vi "GetClassTemplates.vi"(0 "ClassWriterGOOP400 in":refnum<class "ClassWriterGOOP400.lvclass">, 1 "DerivedFromThisClass(if any)":refnum<vi>, 5 "error in (no error)":errorcluster) -> (14 "ClassWriterGOOP400 out":refnum<class "ClassWriterGOOP400.lvclass">, 15 "Templates":T1[](array[typedef]), 19 "error out":errorcluster)   [LabVIEW 2020, in "ClassWriterGOOP400.lvclass"]
uses:
  <resource>/Framework/Providers/Open_GDS/ClassProviders/Provider_EndevoGOOP400/ClassWriterGOOP400_class/ClassWriterGOOP400.lvclass
  <resource>/Framework/Providers/Open_GDS/ClassProviders/Provider_BaseClassInterface/ClassTemplateType.ctl
  <resource>/Framework/Providers/Open_GDS/ClassProviders/Provider_EndevoGOOP400/Templates/EndevoG4TemplateNames.ctl
  <resource>/Framework/Providers/Open_GDS/ClassProviders/Common/ScriptingFunctions/Scripting_ConnectorPanePatternType.ctl
  <resource>/Framework/Providers/Open_GDS/ClassProviders/Provider_BaseClassInterface/ClassWriter_class/ClassWriter.lvclass
  <resource>/Framework/Providers/Open_GDS/ClassProviders/Provider_LvNativeClass/ClassWriterNative_class/ClassWriterNative.lvclass
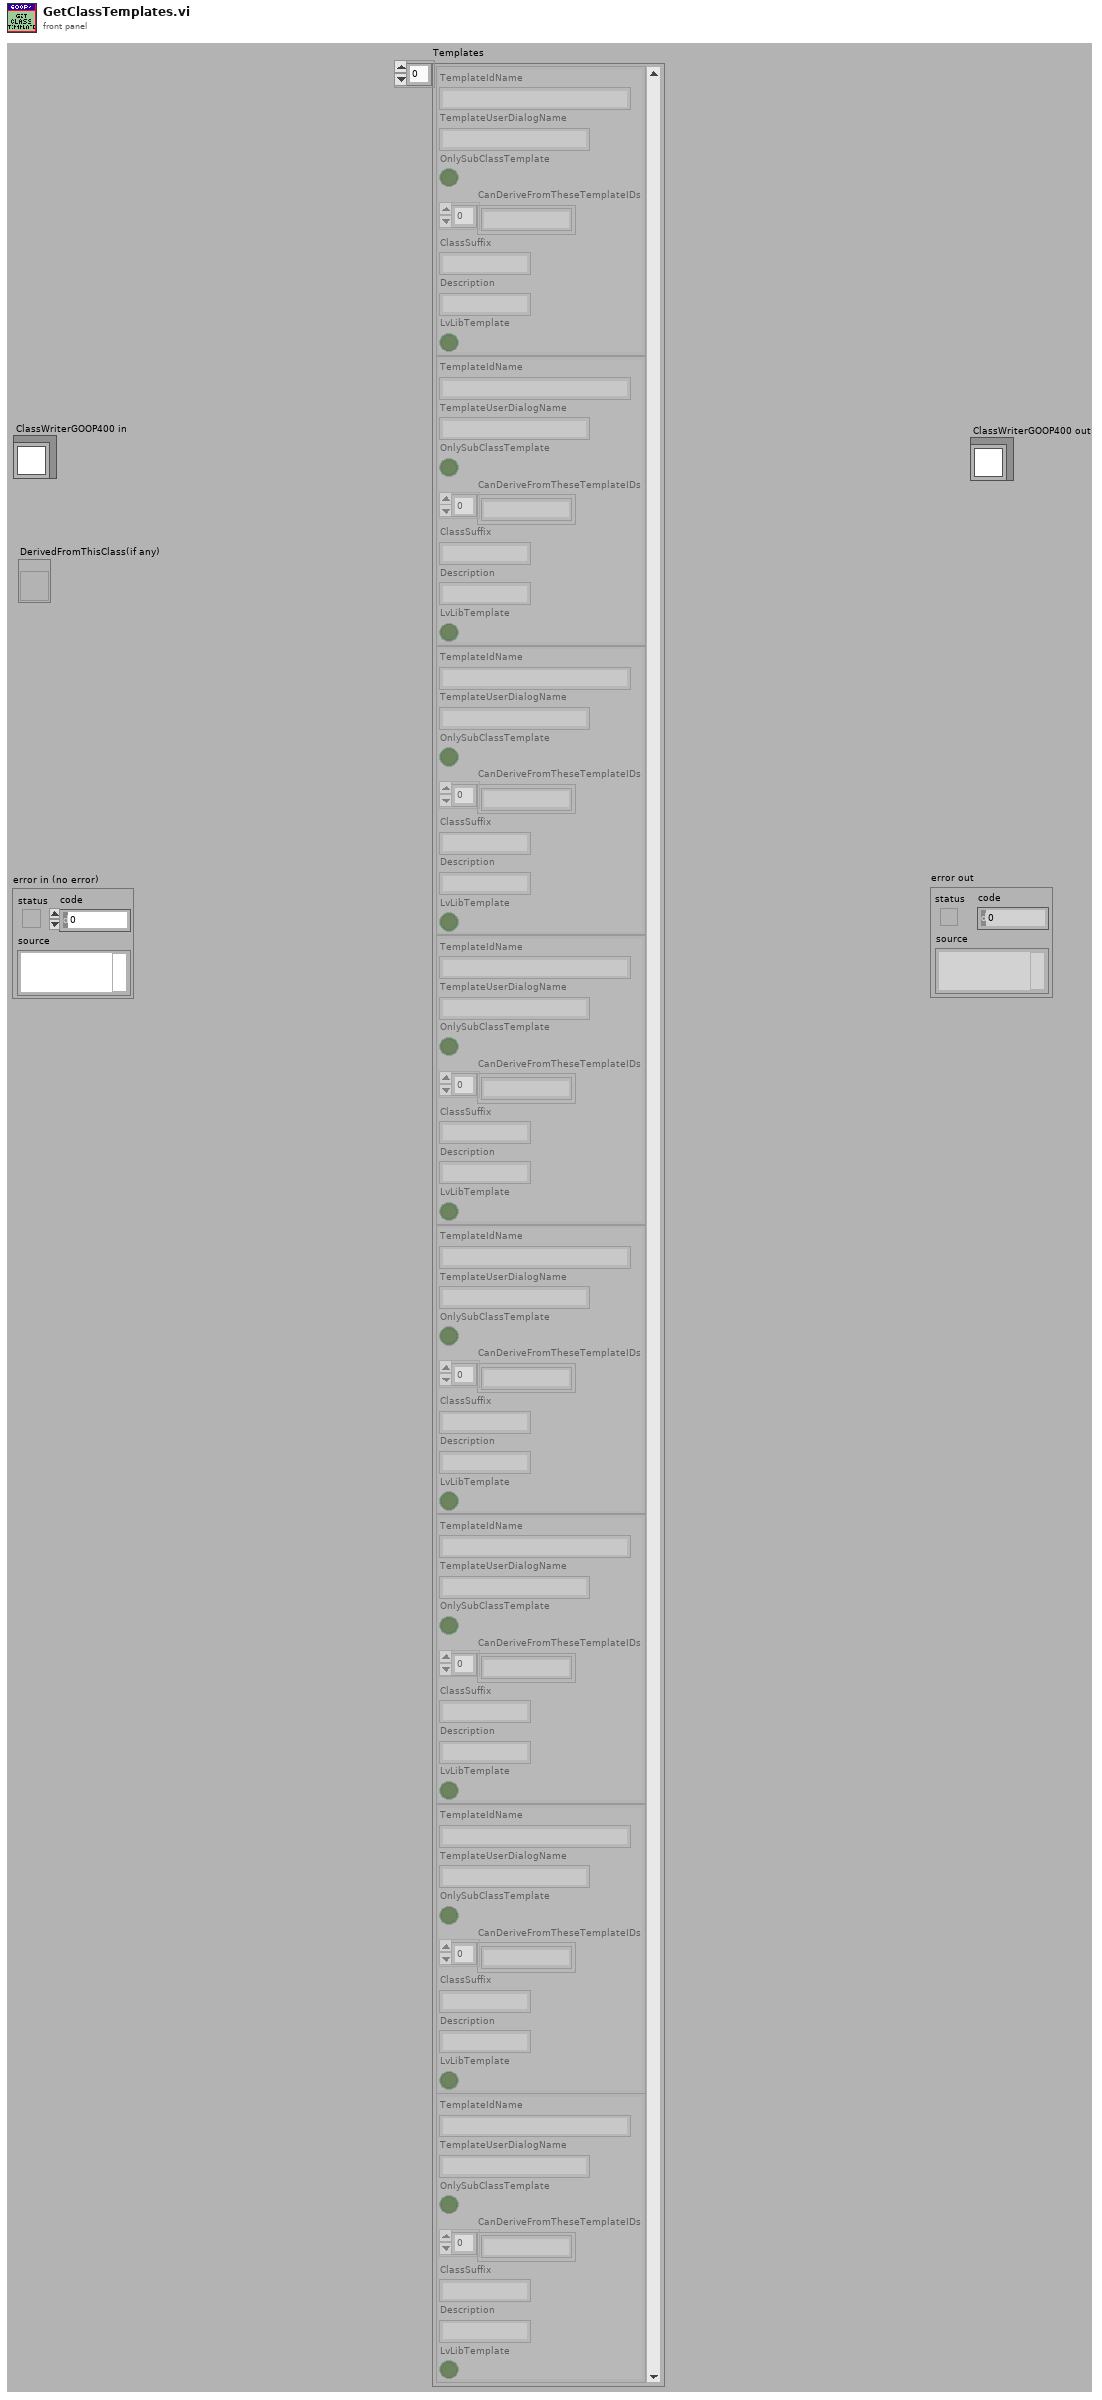
[diagram p1: front panel]
types:
  T1 = typedef "ClassWriter.lvclass/ClassTemplateType.ctl" = cluster{"TemplateIdName":string, "TemplateUserDialogName":string, "OnlySubClassTemplate":bool, "CanDeriveFromTheseTemplateIDs":string[], "ClassSuffix":string, "Description":string, "LvLibTemplate":bool}
  T2 = typedef "EndevoG4TemplateNames.ctl" = enum16{"G4BaseTemplate_Simple_4x4x4", "G4SubTemplate_Simple_4x4x4", "G4BaseTemplate_Simple_6x8x6", "G4SubTemplate_Simple_6x8x6", "G4BaseTemplate_Singleton_4x4x4", "G4SubTemplate_Singleton_4x4x4", "G4BaseTemplate_Singleton_6x8x6", "G4SubTemplate_Singleton_6x8x6", "G4InterfaceTemplate_6x8x6", "G4InterfaceTemplate_4x4x4", "G4BaseTemplate_Simple_5x6x5", "G4BaseTemplate_Singleton_5x6x5", "G4InterfaceTemplate_5x6x5", "G4SubTemplate_Simple_5x6x5", "G4SubTemplate_Singleton_5x6x5"}
  T3 = typedef "Scripting_ConnectorPanePatternType.ctl" = u16
  T4 = typedef "GDSLvCLass_ClassSettingsType.ctl" = cluster{"ClassProviderName":string, "ClassTemplateUsed":string, "ClassTemplateVersion":string, "ClassDescription":string, "PlugIns":T5[], "ConnectorPanePattern":string}
  T5 = typedef "GDSLvClass_PlugIn.ctl" = cluster{"Type":T6, "ID":string, "Version":string, "Path":path, "Name":string, "Data":variant}
  T6 = typedef "GDSLvClass_PlugInTypes.ctl" = enum16{"DesignPattern", "MethodTypes"}
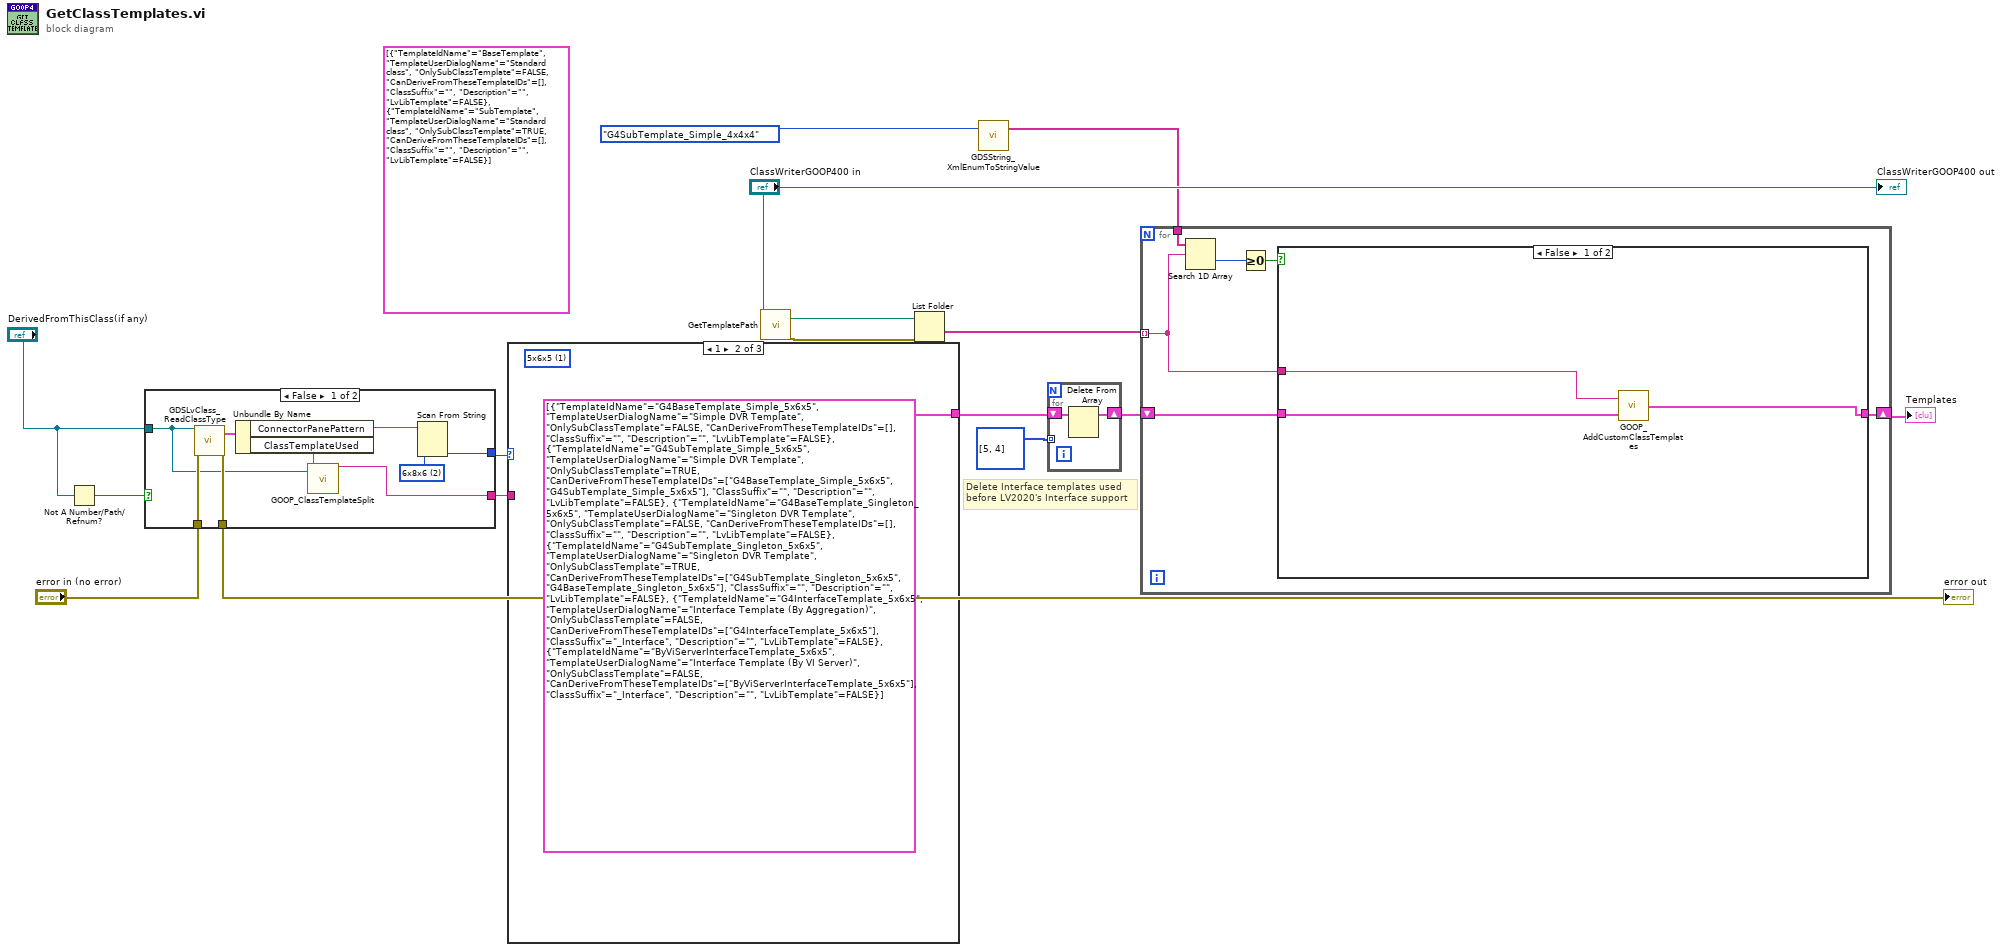
[diagram p0: block diagram]
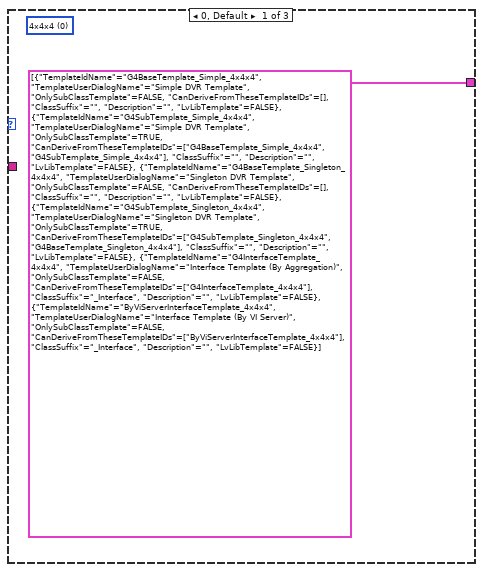
[diagram p2: hidden frame]
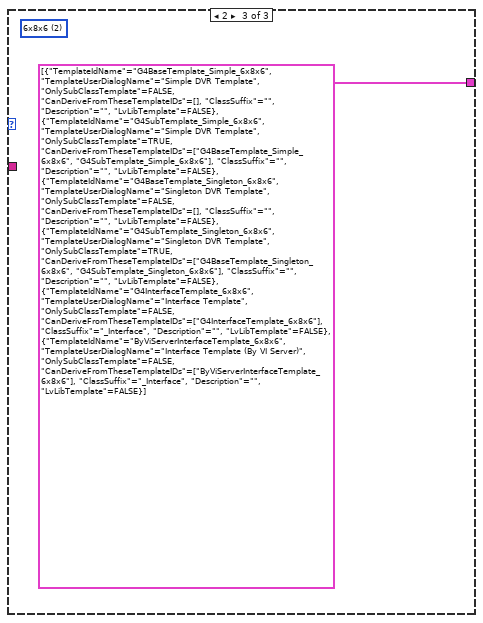
[diagram p3: hidden frame]
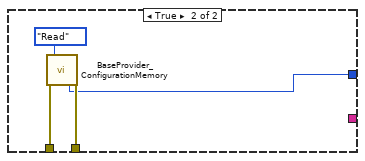
[diagram p4: hidden frame]
diagram:
  (unwired) T1[] [{"TemplateIdName"="BaseTemplate", "TemplateUserDialogName"="Standard class", "OnlySubClassTemplate"=FALSE, "CanDeriveFromTheseTemplateIDs"=[], "ClassSuffix"="", "Description"="", "LvLibTemplate"=FALSE}, {"TemplateIdName"="SubTemplate", "TemplateUserDialogName"="Standard class", "OnlySubClassTemplate"=TRUE, "CanDeriveFromTheseTemplateIDs"=[], "ClassSuffix"="", "Description"="", "LvLibTemplate"=FALSE}] ("TemplateIdNames")
  # "Delete Interface templates used\nbefore LV2020's Interface support"
  n1 = Not A Number/Path/Refnum?(number/path/refnum="DerivedFromThisClass(if any)") -> (NaN/Path/Refnum?=w11:bool)
  n2 = case shown="False" w11 {
    tunnel: "error in (no error)" -> [w22 w28]
    tunnel: "DerivedFromThisClass(if any)" -> [w17 _]
    tunnel: [w21 w27] -> w7
    tunnel: [w20 w26] -> w10
    tunnel: [w18 _] -> w6
    frame False {
      w23 = T3 2 items=["4x4x4", "5x6x5", "6x8x6"] ("Pattern")
      n3 = call <resource>:"GDSLvClass_ReadClassType.vi"("Class Refnum In"=w17, "error in (no error)"=w22) -> ("ClassSettings"=w25:T4, "error out"=w21:errorcluster)  [unwired: 15 in, 1 out]
      n4 = Unbundle By Name(w25) -> ("ConnectorPanePattern"=w24:string, "ClassTemplateUsed"=w19:string)
      n5 = call <resource>:"GOOP_ClassTemplateSplit.vi"("ClassItemRefIn"=w17, "FullClassTemplate"=w19) -> ("StandardTemplate"=w18:string)  [unwired: 12 in, 1 out]
      n6 = Scan From String(input string=w24, default 1=w23) -> (output 1=w20:T3)  [unwired: 3 in, 3 out]
    }
    frame True {
      n7 = call <resource>:"BaseProvider_ConfigurationMemory.vi"("error in (no error)"=w28, "Action"=enum16{"Read", "Load", "Save"}."Read") -> ("PatternOut"=w26:T3, "error out"=w27:errorcluster)  [unwired: 11 in, 5 out]
    }
  }
  "error out" <- w7
  n8 = case shown="1" w10 {
    tunnel: [T1[] [{"TemplateIdName"="G4BaseTemplate_Simple_4x4x4", "TemplateUserDialogName"="Simple DVR Template", "OnlySubClassTemplate"=FALSE, "CanDeriveFromTheseTemplateIDs"=[], "ClassSuffix"="", "Description"="", "LvLibTemplate"=FALSE}, {"TemplateIdName"="G4SubTemplate_Simple_4x4x4", "TemplateUserDialogName"="Simple DVR Template", "OnlySubClassTemplate"=TRUE, "CanDeriveFromTheseTemplateIDs"=["G4BaseTemplate_Simple_4x4x4", "G4SubTemplate_Simple_4x4x4"], "ClassSuffix"="", "Description"="", "LvLibTemplate"=FALSE}, {"TemplateIdName"="G4BaseTemplate_Singleton_4x4x4", "TemplateUserDialogName"="Singleton DVR Template", "OnlySubClassTemplate"=FALSE, "CanDeriveFromTheseTemplateIDs"=[], "ClassSuffix"="", "Description"="", "LvLibTemplate"=FALSE}, {"TemplateIdName"="G4SubTemplate_Singleton_4x4x4", "TemplateUserDialogName"="Singleton DVR Template", "OnlySubClassTemplate"=TRUE, "CanDeriveFromTheseTemplateIDs"=["G4SubTemplate_Singleton_4x4x4", "G4BaseTemplate_Singleton_4x4x4"], "ClassSuffix"="", "Description"="", "LvLibTemplate"=FALSE}, {"TemplateIdName"="G4InterfaceTemplate_4x4x4", "TemplateUserDialogName"="Interface Template (By Aggregation)", "OnlySubClassTemplate"=FALSE, "CanDeriveFromTheseTemplateIDs"=["G4InterfaceTemplate_4x4x4"], "ClassSuffix"="_Interface", "Description"="", "LvLibTemplate"=FALSE}, {"TemplateIdName"="ByViServerInterfaceTemplate_4x4x4", "TemplateUserDialogName"="Interface Template (By VI Server)", "OnlySubClassTemplate"=FALSE, "CanDeriveFromTheseTemplateIDs"=["ByViServerInterfaceTemplate_4x4x4"], "ClassSuffix"="_Interface", "Description"="", "LvLibTemplate"=FALSE}] ("TemplateIdNames") T1[] [{"TemplateIdName"="G4BaseTemplate_Simple_5x6x5", "TemplateUserDialogName"="Simple DVR Template", "OnlySubClassTemplate"=FALSE, "CanDeriveFromTheseTemplateIDs"=[], "ClassSuffix"="", "Description"="", "LvLibTemplate"=FALSE}, {"TemplateIdName"="G4SubTemplate_Simple_5x6x5", "TemplateUserDialogName"="Simple DVR Template", "OnlySubClassTemplate"=TRUE, "CanDeriveFromTheseTemplateIDs"=["G4BaseTemplate_Simple_5x6x5", "G4SubTemplate_Simple_5x6x5"], "ClassSuffix"="", "Description"="", "LvLibTemplate"=FALSE}, {"TemplateIdName"="G4BaseTemplate_Singleton_5x6x5", "TemplateUserDialogName"="Singleton DVR Template", "OnlySubClassTemplate"=FALSE, "CanDeriveFromTheseTemplateIDs"=[], "ClassSuffix"="", "Description"="", "LvLibTemplate"=FALSE}, {"TemplateIdName"="G4SubTemplate_Singleton_5x6x5", "TemplateUserDialogName"="Singleton DVR Template", "OnlySubClassTemplate"=TRUE, "CanDeriveFromTheseTemplateIDs"=["G4SubTemplate_Singleton_5x6x5", "G4BaseTemplate_Singleton_5x6x5"], "ClassSuffix"="", "Description"="", "LvLibTemplate"=FALSE}, {"TemplateIdName"="G4InterfaceTemplate_5x6x5", "TemplateUserDialogName"="Interface Template (By Aggregation)", "OnlySubClassTemplate"=FALSE, "CanDeriveFromTheseTemplateIDs"=["G4InterfaceTemplate_5x6x5"], "ClassSuffix"="_Interface", "Description"="", "LvLibTemplate"=FALSE}, {"TemplateIdName"="ByViServerInterfaceTemplate_5x6x5", "TemplateUserDialogName"="Interface Template (By VI Server)", "OnlySubClassTemplate"=FALSE, "CanDeriveFromTheseTemplateIDs"=["ByViServerInterfaceTemplate_5x6x5"], "ClassSuffix"="_Interface", "Description"="", "LvLibTemplate"=FALSE}] ("TemplateIdNames") T1[] [{"TemplateIdName"="G4BaseTemplate_Simple_6x8x6", "TemplateUserDialogName"="Simple DVR Template", "OnlySubClassTemplate"=FALSE, "CanDeriveFromTheseTemplateIDs"=[], "ClassSuffix"="", "Description"="", "LvLibTemplate"=FALSE}, {"TemplateIdName"="G4SubTemplate_Simple_6x8x6", "TemplateUserDialogName"="Simple DVR Template", "OnlySubClassTemplate"=TRUE, "CanDeriveFromTheseTemplateIDs"=["G4BaseTemplate_Simple_6x8x6", "G4SubTemplate_Simple_6x8x6"], "ClassSuffix"="", "Description"="", "LvLibTemplate"=FALSE}, {"TemplateIdName"="G4BaseTemplate_Singleton_6x8x6", "TemplateUserDialogName"="Singleton DVR Template", "OnlySubClassTemplate"=FALSE, "CanDeriveFromTheseTemplateIDs"=[], "ClassSuffix"="", "Description"="", "LvLibTemplate"=FALSE}, {"TemplateIdName"="G4SubTemplate_Singleton_6x8x6", "TemplateUserDialogName"="Singleton DVR Template", "OnlySubClassTemplate"=TRUE, "CanDeriveFromTheseTemplateIDs"=["G4BaseTemplate_Singleton_6x8x6", "G4SubTemplate_Singleton_6x8x6"], "ClassSuffix"="", "Description"="", "LvLibTemplate"=FALSE}, {"TemplateIdName"="G4InterfaceTemplate_6x8x6", "TemplateUserDialogName"="Interface Template", "OnlySubClassTemplate"=FALSE, "CanDeriveFromTheseTemplateIDs"=["G4InterfaceTemplate_6x8x6"], "ClassSuffix"="_Interface", "Description"="", "LvLibTemplate"=FALSE}, {"TemplateIdName"="ByViServerInterfaceTemplate_6x8x6", "TemplateUserDialogName"="Interface Template (By VI Server)", "OnlySubClassTemplate"=FALSE, "CanDeriveFromTheseTemplateIDs"=["ByViServerInterfaceTemplate_6x8x6"], "ClassSuffix"="_Interface", "Description"="", "LvLibTemplate"=FALSE}] ("TemplateIdNames")] -> w3
    tunnel: w6 -> [_ _ _]
    frame 0, Default {
      (unwired) T3 0 items=["4x4x4", "5x6x5", "6x8x6"] ("Pattern")
    }
    frame 1 {
      (unwired) T3 1 items=["4x4x4", "5x6x5", "6x8x6"] ("Pattern")
    }
    frame 2 {
      (unwired) T3 2 items=["4x4x4", "5x6x5", "6x8x6"] ("Pattern")
    }
  }
  n9 = call-dynamic "GetTemplatePath.vi"("reference in"="ClassWriterGOOP400 in") -> ("FolderPathOut"=w16:path, "error out"=w15:errorcluster)  [unwired: 14 in, 3 out]
  n10 = List Folder(path=w16, error in=w15) -> (folder names=w14:string[])  [unwired: 2 in, 3 out]
  n11 = call <resource>:"GDSString_XmlEnumToStringValue.vi"("EnumVariantIn(used if String is Empty)"=EndevoG4TemplateNames."G4SubTemplate_Simple_4x4x4" ("TemplateNames")) -> ("EnumItems(string)"=w4:string[])  [unwired: 15 in, 3 out]
  n12 = for {
    shift-right: [w33] -> w2
    shift-left: w3 -> [w34]
    tunnel: i32[] [5, 4] ("index") -> [_] mode=indexing
    n13 = Delete From Array(array=w34) -> (array with subset deleted=w33:T1[])  [unwired: 2 in, 1 out]
  }
  n14 = for {
    tunnel: w14 -> [w37] mode=indexing
    shift-right: [w40] -> w13
    shift-left: w2 -> [w39]
    tunnel: w4 -> [w38]
    n15 = Search 1D Array(1D array=w38, element=w37) -> (index of element=w36:i32)  [unwired: 1 in]
    n16 = Greater Or Equal To 0?(x=w36) -> (x >= 0?=w35:bool)
    n17 = case shown="False" w35 {
      tunnel: [w43 w44] -> w40
      tunnel: w39 -> [w42 w44]
      tunnel: w37 -> [w41 _]
      frame False {
        n18 = call <resource>:"GOOP_AddCustomClassTemplates.vi"("TemplateIdNames"=w42, "String"=w41) -> ("TemplateIdNames 2"=w43:T1[])
      }
      frame True {
      }
    }
  }
  "Templates" <- w13
  "ClassWriterGOOP400 out" <- "ClassWriterGOOP400 in"
